vi "Run All Tests in Project.vi"() -> ()   [LabVIEW 2020]
uses:
  Framework/Execution UI/Public/Execution Mode.ctl
  Framework/Execution UI/User Interface.vi
  Framework/Execution UI/Execution UI.lvclass
panel:
  out "error out":errorcluster
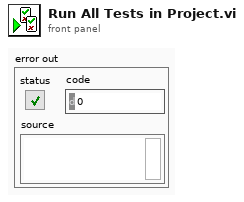
[diagram p1: front panel]
types:
  T1 = enum32{"Invalid", "Standard", "Closed", "Hidden", "Minimized", "Maximized"}
  T2 = typedef "Execution UI.lvclass/Execution Mode.ctl" = enum16{"Default", "Run Tests In Project", "Run Test Case"}
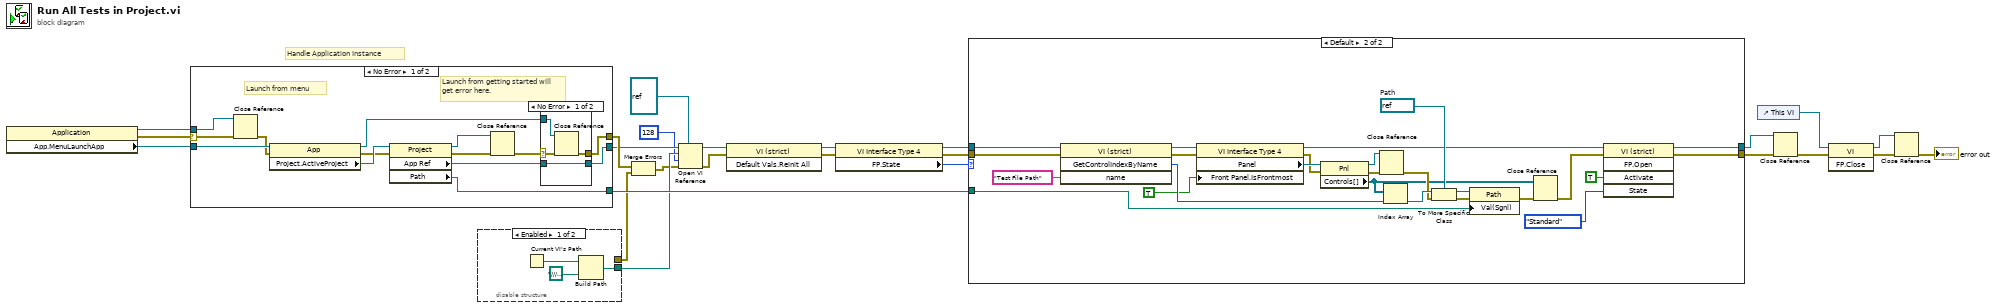
[diagram p0: block diagram]
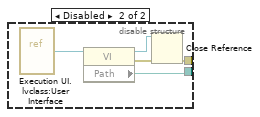
[diagram p2: hidden frame]
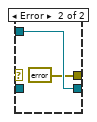
[diagram p3: hidden frame]
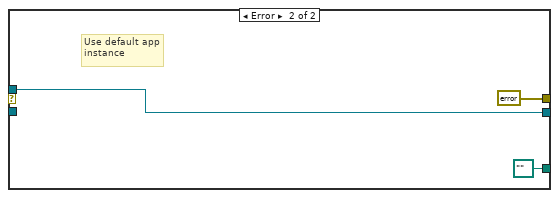
[diagram p4: hidden frame]
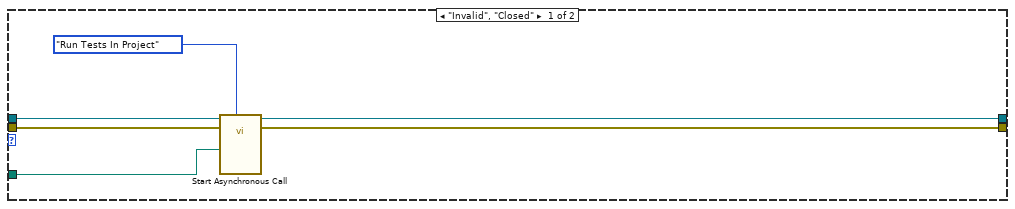
[diagram p5: hidden frame]
diagram:
  # "Handle Application Instance"
  n1 = property class="Application"() -> (reference out=w5:refnum<vi>, error out=w6:errorcluster, "App.MenuLaunchApp"=w7:refnum<vi>)  [unwired: 2 in]
  n2 = case shown="No Error" w6 {
    selector: w6 -> [w38 _]
    tunnel: [w31 w48] -> w11
    tunnel: w7 -> [w36 _]
    tunnel: w5 -> [w39 w48]
    tunnel: [w27 errorcluster {"status"=FALSE, "code"=0, "source"=""} ("error out")] -> w12
    tunnel: [w26 path "" ("Path")] -> w23
    frame No Error {
      # "Launch from getting started will get error here."
      # "Launch from menu"
      n3 = Close Reference(reference=w39, error in (no error)=w38) -> (error out=w35:errorcluster)
      n4 = property class="App"(reference=w36, error in=w35) -> (reference out=w34:refnum<vi>, error out=w32:errorcluster, "Project.ActiveProject"=w37:refnum<vi>)
      n5 = property class="Project"(reference=w37, error in=w32) -> (reference out=w33:refnum<vi>, error out=w29:errorcluster, "App Ref"=w30:refnum<vi>, "Path"=w26:path)
      n6 = Close Reference(reference=w33, error in (no error)=w29) -> (error out=w28:errorcluster)
      n7 = case shown="No Error" w28 {
        selector: w28 -> [w42 _]
        tunnel: w34 -> [w43 w45]
        tunnel: [w41 errorcluster {"status"=FALSE, "code"=0, "source"=""} ("error out")] -> w27
        tunnel: [w40 w45] -> w31
        tunnel: w30 -> [w40 _]
        frame No Error {
          n8 = Close Reference(reference=w43, error in (no error)=w42) -> (error out=w41:errorcluster)
        }
        frame Error {
        }
      }
    }
    frame Error {
      # "Use default app instance"
    }
  }
  n9 = disable-structure shown="Enabled" {
    disable-tunnel: [w51 w53] -> w8
    disable-tunnel: [_ w52] -> w2
    frame Enabled {
      n10 = Current VI's Path() -> (path=w49:path)
      n11 = Build Path(base path=w49, name or relative path=path "../../../vi.lib/Astemes/LUnit/LUnit User Interface.vi") -> (appended path=w51:path)
    }
    frame Disabled {
      n12 = vi-ref "Execution UI.lvclass:User Interface.vi"() -> (w56:refnum<vi>)
      n13 = property class="VI"(reference=w56) -> (reference out=w55:refnum<vi>, error out=w54:errorcluster, "Path"=w53:path)  [unwired: 1 in]
      n14 = Close Reference(reference=w55, error in (no error)=w54) -> (error out=w52:errorcluster)
    }
  }
  n15 = Merge Errors(w12, w2) -> (w3:errorcluster)
  n16 = Open VI Reference(type specifier VI Refnum (for type only)=refnum<vi> refnum, application reference (local)=w11, vi path=w8, options=128, error in (no error)=w3) -> (vi reference=w10:refnum<vi>, error out=w9:errorcluster)  [unwired: 1 in]
  n17 = invoke class="VI (strict)" method="Default Vals.Reinit All"(reference=w10, error in=w9) -> (reference out=w22:refnum<vi>, error out=w19:errorcluster)  [unwired: 1 in, 1 out]
  n18 = property class="VI Interface Type 4"(reference=w22, error in=w19) -> (reference out=w20:refnum<vi>, error out=w21:errorcluster, "FP.State"=w18:T1)
  n19 = case shown="Default" w18 {
    tunnel: [w62 w68] -> w25
    tunnel: w23 -> [w61 w74]
    tunnel: [w59 w69] -> w24
    tunnel: w20 -> [w58 w76]
    tunnel: w21 -> [w57 w75]
    frame "Invalid", "Closed" {
      n20 = call-by-ref "Start Asynchronous Call"(reference=w58, error in=w57, "Execution Mode"=Execution_Mode."Run Tests In Project", "Test File Path"=w61) -> (reference out=w59:refnum<vi>, error out=w62:errorcluster)  [unwired: 10 in]
    }
    frame Default {
      w83 = refnum<vi> refnum  # Path
      n21 = invoke class="VI (strict)" method="GetControlIndexByName"(reference=w76, error in=w75, "name"="Test File Path" ("Control Name")) -> (reference out=w86:refnum<vi>, error out=w77:errorcluster, "GetControlIndexByName"=w84:i32)  [unwired: 1 in, 1 out]
      n22 = property class="VI Interface Type 4"(reference=w86, error in=w77, "Front Panel.IsFrontmost"=TRUE ("Front Panel Window:Is Frontmost")) -> (reference out=w70:refnum<vi>, error out=w78:errorcluster, "Panel"=w87:refnum<vi>)
      n23 = property class="Pnl"(reference=w87, error in=w78) -> (reference out=w71:refnum<vi>, error out=w79:errorcluster, "Controls[]"=w63:refnum<vi>[])
      n24 = Close Reference(reference=w71, error in (no error)=w79) -> (error out=w72:errorcluster)
      n25 = Index Array(array=w63, index=w84) -> (element=w81:refnum<vi>)
      n26 = To More Specific Class(target class=w83, reference=w81, error in=w72) -> (specific class reference=w82:refnum<vi>, error out=w80:errorcluster)
      n27 = property class="Path"(reference=w82, error in=w80, "Val(Sgnl)"=w74) -> (error out=w73:errorcluster)  [unwired: 1 out]
      n28 = Close Reference(reference=w63, error in (no error)=w73) -> (error out=w67:errorcluster)
      n29 = invoke class="VI (strict)" method="FP.Open"(reference=w70, error in=w67, "Activate"=TRUE ("Activate?"), "State"=T1."Standard") -> (reference out=w69:refnum<vi>, error out=w68:errorcluster)  [unwired: 1 in, 3 out]
    }
  }
  n30 = control-ref of="This VI"() -> (w17:refnum<vi>)
  n31 = Close Reference(reference=w24, error in (no error)=w25) -> (error out=w14:errorcluster)
  n32 = invoke class="VI" method="FP.Close"(reference=w17, error in=w14) -> (reference out=w15:refnum<vi>, error out=w16:errorcluster)  [unwired: 1 in, 1 out]
  n33 = Close Reference(reference=w15, error in (no error)=w16) -> (error out=→"error out":errorcluster)
